vi "Start Module.vi"(6 "Show Main VI Diagram on Init (F)":bool, 8 "error in":errorcluster, 11 "Run as Singleton? (F)":bool) -> (0 "error out":errorcluster, 1 "Wait for Event Sync?":bool, 2 "My Cloneable Module Broadcast Events":T1, 3 "Module ID":i32, 4 "Module Name":string)   [LabVIEW 2025, in "My Cloneable Module.lvlib"]
doc: "Launches an instance of the module Main VI. After calling this VI, you can optionally register for broadcast events from the module by wiring the broadcast events output of this VI to a <b>Register For Events</b> function. \n\nAfter the optional Register For Events function call, you should always call the <b>Synchronize Module Events.vi</b> for this module with the 'Wait for Event Sync?' output of this VI to the corresponding input of the Synchronize Module Events.vi. \n\nTo see an example of the proper wiring pattern, see the \"Run New Module: Value Change\" event frame in the API Tester VI for this module.\n\nThe <b>Validate DQMH Module</b> tool added a 'Module Name' output to this VI.\n_____\nBased on DQMH Dev Tools: Project Template 7.1.0.1503."
uses:
  My Cloneable Module.lvlib
  Broadcast Events--cluster.ctl
  Did Init Argument--cluster.ctl
  Status Updated Argument--cluster.ctl
  Error Reported Argument--cluster.ctl
  Do Something Argument--cluster.ctl
  Stop Argument--cluster.ctl
  Get Module Execution Status Argument--cluster.ctl
  Module Running State--enum.ctl
  <vilib>/Delacor/Delacor QMH/Libraries/Cloneable Module Admin_class/Delacor_lib_QMH_Cloneable Module Admin.lvclass
  C:/Program Files (x86)/National Instruments/LabVIEW 2025/vi.lib/Delacor/Delacor QMH/Libraries/Module Admin_class/Delacor_lib_QMH_Module Admin.lvclass
  VI Reference Management/Main VI Type--strict_vi_ref.ctl
  <vilib>/Delacor/Delacor QMH/Libraries/Cloneable Module Admin_class/Delacor_lib_QMH_Cloneable Module Admin.lvclass/Delacor_lib_QMH_Cloneable Module Admin.ctl
  <vilib>/Delacor/Delacor QMH/Libraries/Module Admin_class/Delacor_lib_QMH_Module Admin.lvclass/Delacor_lib_QMH_Module Admin.ctl
  <vilib>/Delacor/Delacor QMH/Libraries/Cloneable Module Admin_class/Delacor_lib_QMH_Set Module ID.vi
  <vilib>/Delacor/Delacor QMH/Libraries/Module Admin_class/Delacor_lib_QMH_Set External Launch.vi
  Main.vi
  Clone Registration/Clone Registration.lvlib
  VI Reference Management/VI Reference Management.lvlib
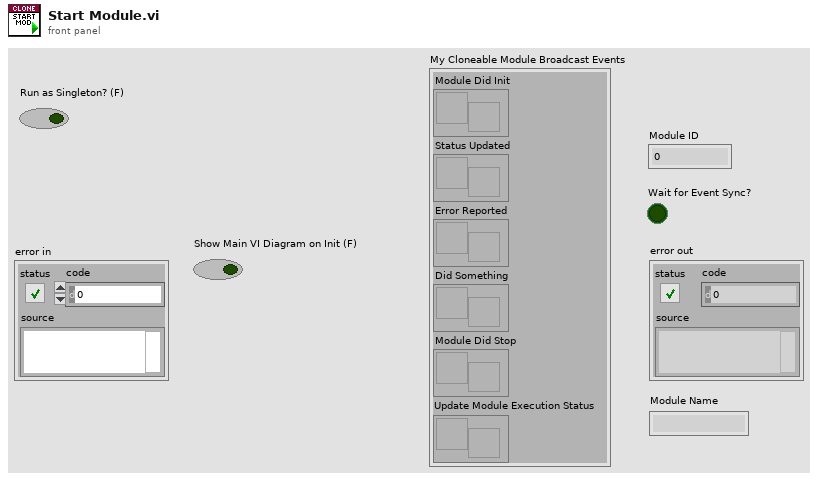
[diagram p1: front panel]
types:
  T1 = typedef "My Cloneable Module.lvlib/Broadcast Events--cluster.ctl" = cluster{"Module Did Init":refnum<user-event>, "Status Updated":refnum<user-event>, "Error Reported":refnum<user-event>, "Did Something":refnum<user-event>, "Module Did Stop":refnum<user-event>, "Update Module Execution Status":refnum<user-event>}
  T2 = typedef "My Cloneable Module.lvlib/Module Running State--enum.ctl" = enum16{"Not Running", "Running as Cloneable", "Running as Singleton"}
  T3 = enum32{"Bad", "Idle", "Run top level", "Running"}
  T4 = typedef "My Cloneable Module.lvlib/VI Reference Management.lvlib/Main VI Type--strict_vi_ref.ctl" = refnum<vi>
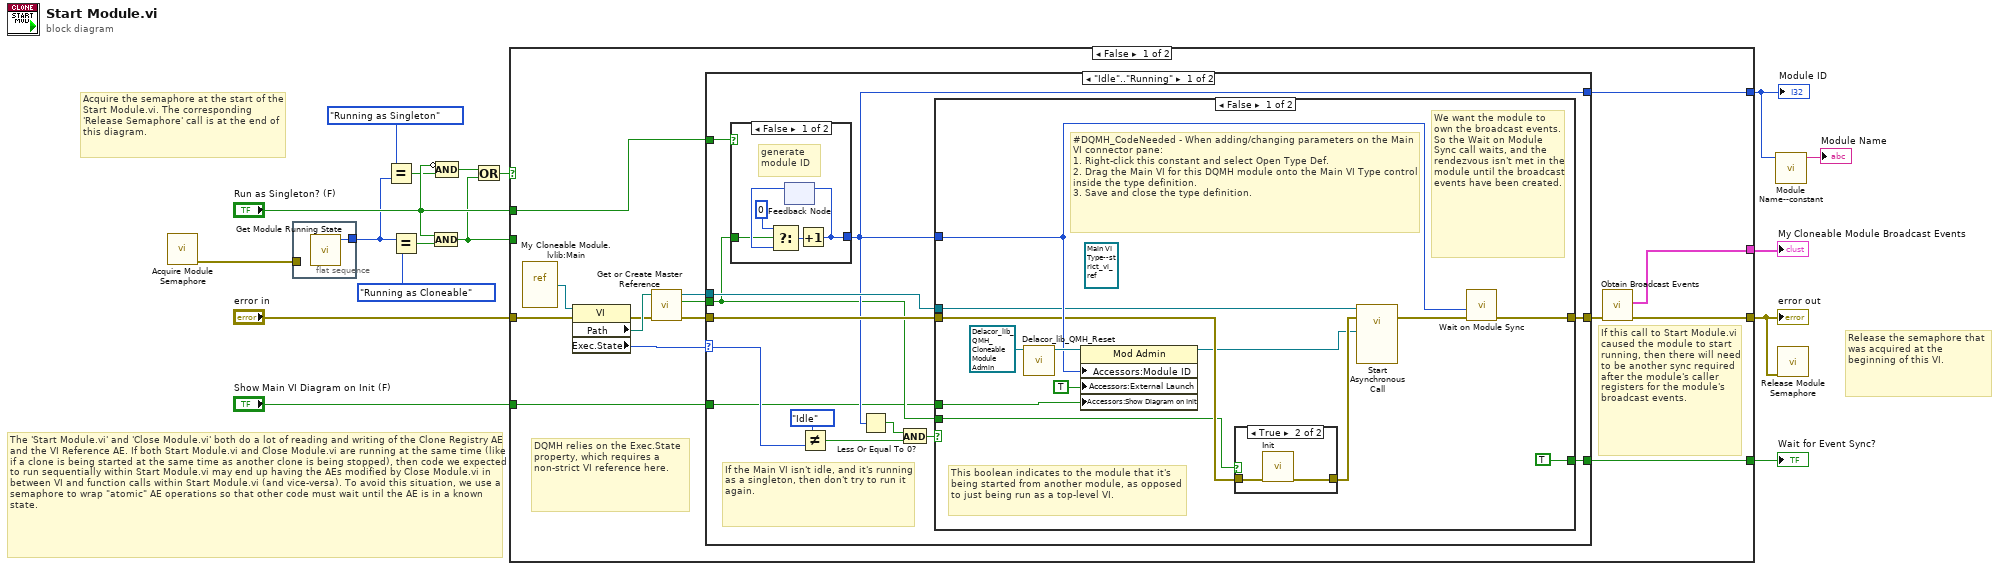
[diagram p0: block diagram]
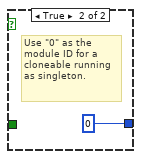
[diagram p2: hidden frame]
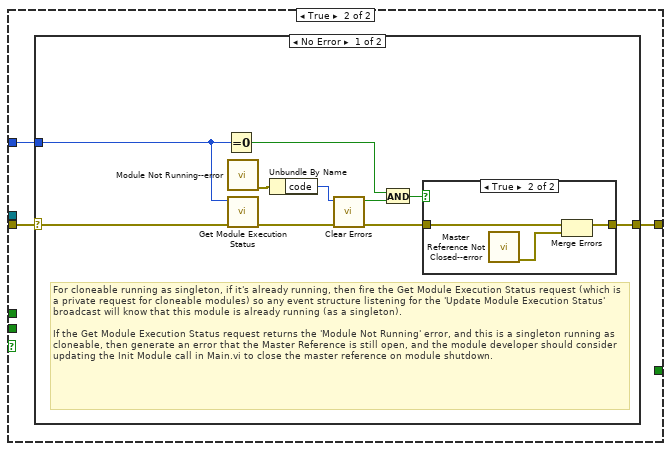
[diagram p4: hidden frame]
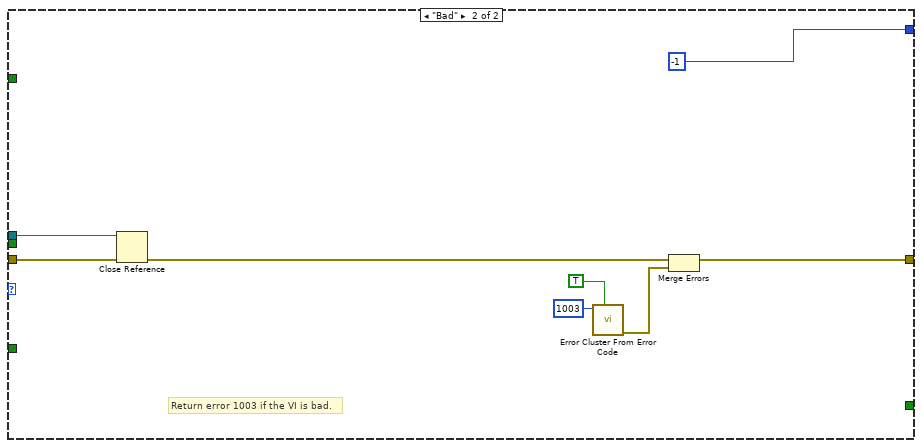
[diagram p7: hidden frame]
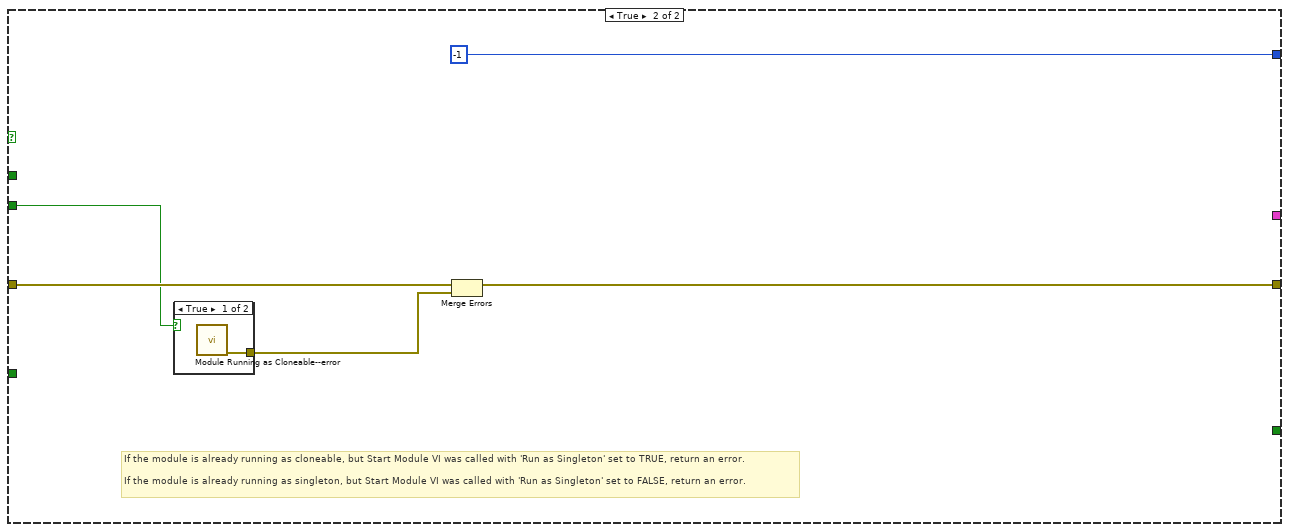
[diagram p8: hidden frame]
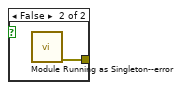
[diagram p9: hidden frame]
diagram:
  # "Release the semaphore that was acquired at the beginning of this VI."
  # "The 'Start Module.vi' and 'Close Module.vi' both do a lot of reading and writing of the Clone Registry AE and the VI Reference AE. If both Start Module.vi and Close Module.vi are running at the same time (like if a clone is being started at the same time as another clone is being stopped), then code we expected to run sequentially within Start Module.vi may end up having the AEs modified by Close Module.vi in between VI and function calls within Start Module.vi (and vice-versa). To avoid this situation, we use a semaphore to wrap \"atomic\" AE operations so that other code must wait until the AE is in a known state."
  # "Acquire the semaphore at the start of the Start Module.vi. The corresponding 'Release Semaphore' call is at the end of this diagram."
  n1 = call "Acquire Module Semaphore.vi"() -> ("error out"=w4:errorcluster)  [unwired: 11 in]
  n2 = flat-sequence {
    tunnel: [w18] -> w7
    tunnel: w4 -> [_]
    frame #0 {
      n3 = call "Get Module Running State.vi"() -> ("Module Running State"=w18:T2)  [unwired: 11 in]
    }
  }
  n4 = Equal?(x=Module_Running_State--enum."Running as Singleton", y=w7) -> (x = y?=w8:bool)
  n5 = Equal?(x=w7, y=Module_Running_State--enum."Running as Cloneable") -> (x = y?=w12:bool)
  n6 = And(x="Run as Singleton? (F)", y=w12) -> (x .and. y?=w5:bool)
  n7 = Compound Arithmetic op=AND(invert "Run as Singleton? (F)", w8) -> (w10:bool)
  n8 = Or(x=w10, y=w5) -> (x .or. y?=w11:bool)
  n9 = case shown="False" w11 {
    tunnel: "error in" -> [w33 w99]
    tunnel: [w31 w98] -> w3
    tunnel: [w30 _] -> w16
    tunnel: [w29 _] -> w15
    tunnel: [w25 -1] -> w14
    tunnel: "Run as Singleton? (F)" -> [w21 _]
    tunnel: w5 -> [_ w95]
    tunnel: "Show Main VI Diagram on Init (F)" -> [w19 _]
    frame False {
      # "DQMH relies on the Exec.State property, which requires a non-strict VI reference here."
      # "If this call to Start Module.vi caused the module to start running, then there will need to be another sync required after the module's caller registers for the module's broadcast events."
      n10 = vi-ref "My Cloneable Module.lvlib:Main.vi"() -> (w24:refnum<vi>)
      n11 = property class="VI"(reference=w24, error in=w33) -> (error out=w27:errorcluster, "Path"=w28:path, "Exec.State"=w22:T3)  [unwired: 1 out]
      n12 = call "Get or Create Master Reference.vi"("error in"=w27, "Main VI Path"=w28) -> ("error out"=w26:errorcluster, "New Reference Created"=w20:bool, "Master Reference"=w23:T4)  [unwired: 7 in]
      n13 = case shown="\"Idle\"..\"Running\"" w22 {
        selector: w22 -> [w42 _]
        tunnel: w26 -> [w46 w94]
        tunnel: w23 -> [w44 w93]
        tunnel: [w43 w91] -> w32
        tunnel: [w45 _] -> w29
        tunnel: [w37 -1] -> w25
        tunnel: w21 -> [w36 _]
        tunnel: w20 -> [w35 _]
        tunnel: w19 -> [w34 _]
        frame "Idle".."Running" {
          # "If the Main VI isn't idle, and it's running as a singleton, then don't try to run it again."
          n14 = case shown="False" w36 {
            tunnel: [w51 0] -> w37
            tunnel: w35 -> [w47 _]
            frame False {
              # "generate module ID"
              n15 = feedback #1() -> (w49:i32)  [unwired: 1 in]
              n16 = Select(t=0, s=w47, f=w49) -> (s? t:f=w50:i32)
              n17 = Increment(x=w50) -> (x+1=w51:i32)
              n18 = feedback-in #1(w51) -> ()
            }
            frame True {
              # "Use \"0\" as the module ID for a cloneable running as singleton."
            }
          }
          n19 = Not Equal?(x=T3."Idle", y=w42) -> (x != y?=w40:bool)
          n20 = Less Or Equal To 0?(x=w37) -> (x <= 0?=w38:bool)
          n21 = And(x=w38, y=w40) -> (x .and. y?=w39:bool)
          n22 = case shown="False" w39 {
            tunnel: w46 -> [w57 w70]
            tunnel: [TRUE _] -> w45
            tunnel: w44 -> [w56 _]
            tunnel: [w60 w69] -> w43
            tunnel: w37 -> [w61 w71]
            tunnel: w35 -> [w54 _]
            tunnel: w34 -> [w53 _]
            frame False {
              (unwired) T4 refnum ("Main VI Type")
              # "#DQMH_CodeNeeded - When adding/changing parameters on the Main VI connector pane:\n1. Right-click this constant and select Open Type Def.\n2. Drag the Main VI for this DQMH module onto the Main VI Type control inside the type definition.\n3. Save and close the type definition."
              # "We want the module to own the broadcast events. So the Wait on Module Sync call waits, and the rendezvous isn't met in the module until the broadcast events have been created."
              # "This boolean indicates to the module that it's being started from another module, as opposed to just being run as a top-level VI."
              n23 = call-dynamic "Delacor_lib_QMH_Reset.vi"("Mod Admin in"=refnum<class "Delacor_lib_QMH_Cloneable Module Admin.lvclass"> refnum) -> ("Mod Admin out"=w64:refnum<class "Delacor_lib_QMH_Cloneable Module Admin.lvclass">)  [unwired: 9 in, 1 out]
              n24 = property class="Mod Admin"(reference=w64, "Accessors:Module ID"=w61, "Accessors:External Launch"=TRUE, "Accessors:Show Diagram on Init"=w53) -> (reference out=w55:refnum<class "Delacor_lib_QMH_Cloneable Module Admin.lvclass">)  [unwired: 1 in, 1 out]
              n25 = case shown="True" w54 {
                tunnel: [w66 w68] -> w58
                tunnel: w57 -> [w66 w67]
                frame False {
                }
                frame True {
                  n26 = call "Init.vi"("error in"=w67) -> ("error out"=w68:errorcluster)  [unwired: 7 in, 3 out]
                }
              }
              n27 = call-by-ref "Start Asynchronous Call"(reference=w56, error in=w58, "Module Admin"=w55) -> (error out=w59:errorcluster)  [unwired: 11 in, 1 out]
              n28 = call "Wait on Module Sync.vi"("error in"=w59, "Module ID"=w61) -> ("error out"=w60:errorcluster)  [unwired: 9 in]
            }
            frame True {
              n29 = case shown="No Error" w70 {
                selector: w70 -> [w81 w86]
                tunnel: w71 -> [w79 _]
                tunnel: [w72 w86] -> w69
                frame No Error {
                  # "For cloneable running as singleton, if it's already running, then fire the Get Module Execution Status request (which is a private request for cloneable modules) so any event structure listening for the 'Update Module Execution Status' broadcast will know that this module is already running (as a singleton).\n\nIf the Get Module Execution Status request returns the 'Module Not Running' error, and this is a singleton running as cloneable, then generate an error that the Master Reference is still open, and the module developer should consider updating the Init Module call in Main.vi to close the master reference on module shutdown."
                  n30 = Equal To 0?(x=w79) -> (x = 0?=w75:bool)
                  n31 = call "Module Not Running--error.vi"() -> ("error out"=w78:errorcluster)  [unwired: 11 in]
                  n32 = call "Get Module Execution Status.vi"("error in"=w81, "Module ID"=w79) -> ("error out"=w80:errorcluster)  [unwired: 9 in]
                  n33 = Unbundle By Name(w78) -> ("code"=w77:i32)
                  n34 = call <vilib>:"Clear Errors.vi"("error in (no error)"=w80, "specific error code to clear (0: all)"=w77) -> ("error out"=w74:errorcluster, "specific error cleared?"=w76:bool)  [unwired: 4 in]
                  n35 = And(x=w75, y=w76) -> (x .and. y?=w73:bool)
                  n36 = case shown="True" w73 {
                    tunnel: w74 -> [w82 w85]
                    tunnel: [w82 w83] -> w72
                    frame False {
                    }
                    frame True {
                      n37 = call "Master Reference Not Closed--error.vi"() -> ("error out"=w84:errorcluster)  [unwired: 11 in]
                      n38 = Merge Errors(w85, w84) -> (w83:errorcluster)
                    }
                  }
                }
                frame Error {
                }
              }
            }
          }
        }
        frame "Bad" {
          # "Return error 1003 if the VI is bad."
          n39 = Close Reference(reference=w93, error in (no error)=w94) -> (error out=w92:errorcluster)
          n40 = call <vilib>:"Error Cluster From Error Code.vi"("show call chain? (False)"=TRUE, "error code (0)"=1003) -> ("error out"=w89:errorcluster)  [unwired: 7 in]
          n41 = Merge Errors(w92, w89) -> (w91:errorcluster)
        }
      }
      n42 = call "Obtain Broadcast Events.vi"("error in"=w32) -> ("error out"=w31:errorcluster, "My Cloneable Module Broadcast Events"=w30:T1)  [unwired: 9 in]
    }
    frame True {
      # "If the module is already running as cloneable, but Start Module VI was called with 'Run as Singleton' set to TRUE, return an error.\n\nIf the module is already running as singleton, but Start Module VI was called with 'Run as Singleton' set to FALSE, return an error."
      n43 = case shown="True" w95 {
        tunnel: [w100 w101] -> w96
        frame True {
          n44 = call "Module Running as Cloneable--error.vi"() -> ("error out"=w100:errorcluster)  [unwired: 11 in]
        }
        frame False {
          n45 = call "Module Running as Singleton--error.vi"() -> ("error out"=w101:errorcluster)  [unwired: 11 in]
        }
      }
      n46 = Merge Errors(w99, w96) -> (w98:errorcluster)
    }
  }
  "error out" <- w3
  "My Cloneable Module Broadcast Events" <- w16
  "Wait for Event Sync?" <- w15
  "Module ID" <- w14
  n47 = call "Module Name--constant.vi"("Module ID"=w14) -> ("Module Name"=→"Module Name":string)  [unwired: 10 in]
  n48 = call "Release Module Semaphore.vi"("error in"=w3) -> ()  [unwired: 10 in, 1 out]
